vi "checkTemperatureSettled.vi"(8 "error in (no error)":errorcluster, 11 "TestMonitor in":refnum<class "TestMonitor.lvclass">) -> (0 "error out":errorcluster, 2 "temperatureSettledIsTrue":bool, 3 "TestMonitor out":refnum<class "TestMonitor.lvclass">)   [LabVIEW 2013, in "TestMonitor.lvclass"]
uses:
  TestMonitor.lvclass
  TestMonitor.lvclass/TestMonitor.ctl
  <vilib>/Analysis/NI_AALBase.lvlib
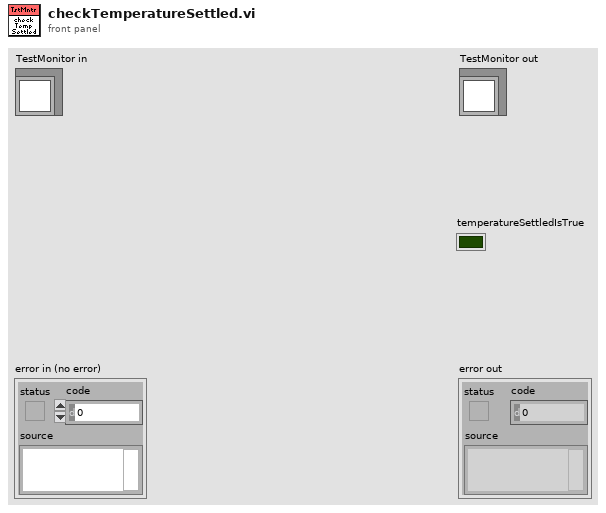
[diagram p1: front panel]
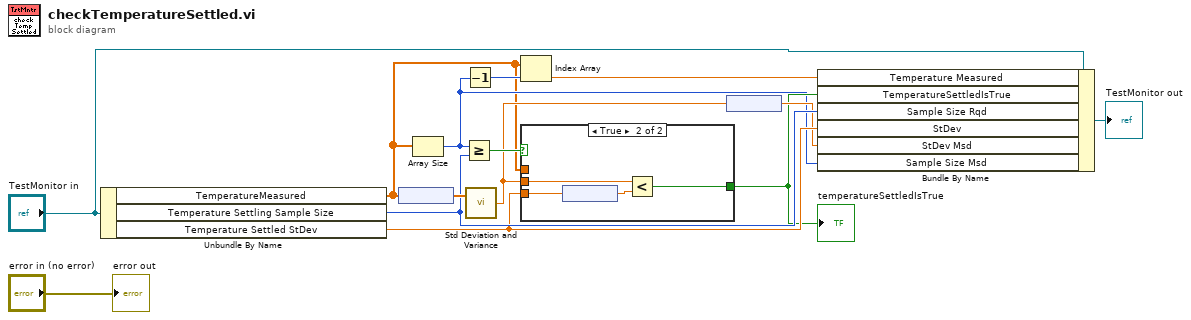
[diagram p0: block diagram]
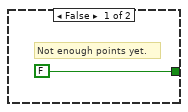
[diagram p2: hidden frame]
diagram:
  n1 = Unbundle By Name("TestMonitor in") -> ("TemperatureMeasured"=w2:dbl[unit][], "Temperature Settling Sample Size"=w9:u16, "Temperature Settled StDev"=w8:dbl[unit])
  n2 = node(w2) -> (w12:dbl[])
  n3 = Array Size(array=w2) -> (size(s)=w3:i32)
  n4 = Greater Or Equal?(x=w3, y=w9) -> (x >= y?=w13:bool)
  n5 = Decrement(x=w3) -> (x-1=w4:i32)
  n6 = call <vilib>:"Std Deviation and Variance.vi"("X"=w12) -> ("standard deviation"=w7:dbl)  [unwired: 1 in, 2 out]
  n7 = Index Array(array=w2, index=w4) -> (element=w1:dbl[unit])
  n8 = case shown="True" w13 {
    tunnel: [FALSE w17] -> w5
    tunnel: w2 -> [_ _]
    tunnel: w8 -> [_ w19]
    tunnel: w7 -> [_ w16]
    frame False {
      # "Not enough points yet."
    }
    frame True {
      n9 = node(w19) -> (w18:dbl)
      n10 = Less?(x=w16, y=w18) -> (x < y?=w17:bool)
    }
  }
  "temperatureSettledIsTrue" <- w5
  n11 = node(w7) -> (w6:dbl[unit])
  n12 = Bundle By Name(cluster="TestMonitor in", "Temperature Measured"=w1, "TemperatureSettledIsTrue"=w5, "Sample Size Rqd"=w9, "StDev"=w8, "StDev Msd"=w6, "Sample Size Msd"=w3) -> (→"TestMonitor out":refnum<class "TestMonitor.lvclass">)
  "error out" <- "error in (no error)"
